vi "Old - Move Straight.vi"(6 "Angle Reduction Factor":dbl, 8 "error in (no error)":errorcluster, 9 "Encoder Reduction Factor":dbl, 10 "Ref-Nums":T1, 11 "Encoder Distance":dbl=-3600.0 format="%#_13g") -> (0 "error out":errorcluster)   [LabVIEW 2017]
uses:
  <vilib>/Rock Robotics/WPI/ThirdParty/Phoenix-LabVIEW/Motor Controller/Get/CTRE_Phoenix_MotorController_GetGeneralStatus.vi
  <vilib>/Rock Robotics/WPI/ThirdParty/Phoenix-LabVIEW/Motor Controller/Get/CTRE_Phoenix_MotorController_GetOutputCurrent_Enhanced.vi
panel:
  in  "Reduction Factor 3":dbl
  in  "Encoder Distance 3":dbl=-3600.0 format="%#_13g"
  in  "Reduction Factor 2":dbl
  in  "Encoder Distance 2":dbl=-3600.0 format="%#_13g"
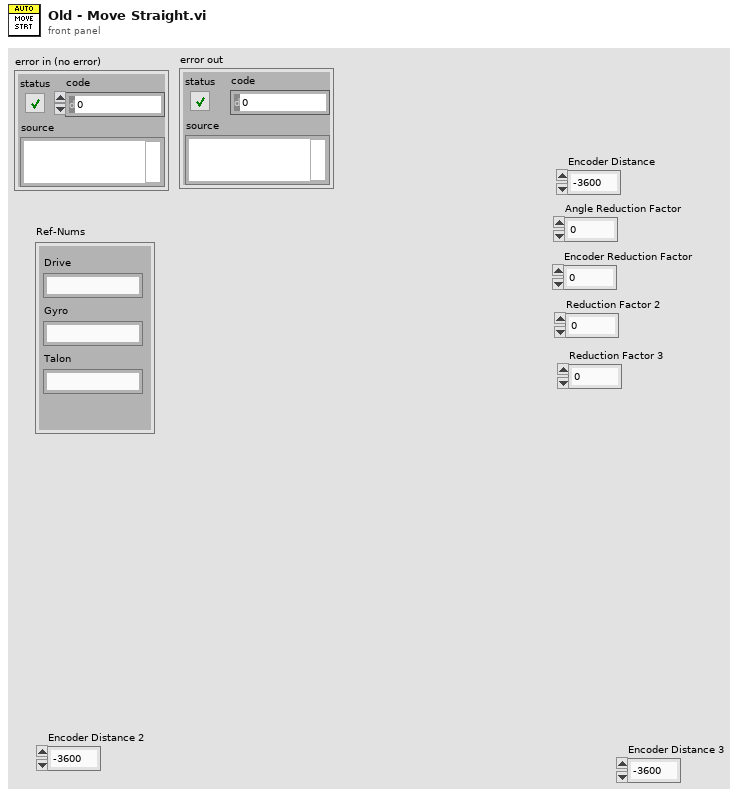
[diagram p1: front panel]
types:
  T1 = cluster{"Drive":string, "Gyro":string, "Talon":string}
  T2 = typedef "WPI_CANTalonSRX_GlobalStatus.ctl" = cluster{"Applied Throttle":dbl, "Module Enabled":bool, "CAN Error":errorcluster, "Closed Loop Error":dbl, "Forward Limit Switch Closed":bool, "Reverse Limit Switch Closed":bool, "Sensor Position":dbl, "Sensor Velocity":dbl, "Current":dbl, "Sticky Fault - Over Temp":bool, "Sticky Fault - Under Voltage":bool, "Sticky Fault - Forward Limit":bool, "Sticky Fault - Reverse Limit":bool, "Sticky Fault - Forward Soft Limit":bool, "Sticky Fault - Reverse Soft Limit":bool, "Brake is Enabled":bool, "Encoder Position":dbl, "Encoder Velocity":dbl, "Encoder Index Count":dbl, "Encoder A Pin State":bool, "Encoder B Pin State":bool, "Encoder Index Pin State":bool, "Analog In":dbl, "Analog In Velocity":dbl, "Temperature (C)":dbl, "Battery Voltage":dbl, "Control 5 Is Supported":bool, "Current Profile Slot Select":dbl, "Pos Div 8":bool, "Vel Div 4":bool, "Pulse Width Position":i32, "Pulse Width Velocity":i32, "Pulse Width Rise To Rise (us)":i32, "Pulse Width Rise To Fall (us)":i32, "Mot Prof Active Is Under Run":bool, "Mot Prof Active Has Under Run":bool, "Mot Prof Active Is Last":bool, "Mot Prof Active Velocity Only":bool, "Mot Prof Active Is Valid":bool, "Mot Prof Buffer Is Full":bool, "Mot Prof Active Profile Slot Select":i32, "Mot Prof NextID":i32, "Mot Prof Count":i32, "Mot Prof Active Velocity":dbl, "Mot Prof Active Position":dbl, "Mot Prof Output Enable":i32}
  T3 = typedef "WPI_MotorControlDeviceRef.ctl" = cluster{"DeviceStatus":errorcluster, "Type":T4, "PWM":cluster{"PWM Channel":T5, "DeadBand":T6}, "CAN":cluster{"Device Number":u8, "SetOutput VI Ref":variant, "GetOutput VI Ref":variant, "Enable VI Ref":variant, "Disable VI Ref":variant, "Data":variant}, "Invert":bool, "DIO PWM":cluster{"PWM \"Enable\" Channel":T5, "DIOChannel":T7, "PWM Rate":dbl}}
  T4 = typedef "WPI_MotorControlType.ctl" = enum16{"PWM", "CAN", "DIO PWM"}
  T5 = typedef "FPGA_DIOPWMChannel.ctl" = enum8{"PWM 0", "PWM 1", "PWM 2", "PWM 3", "PWM 4", "PWM 5", "PWM 6", "PWM 7", "PWM 8", "PWM 9", "PWM MXP 0", "PWM MXP 1", "PWM MXP 2", "PWM MXP 3", "PWM MXP 4", "PWM MXP 5", "PWM MXP 6", "PWM MXP 7", "PWM MXP 8", "PWM MXP 9", "Invalid"}
  T6 = typedef "WPI_PWMDeadband.ctl" = cluster{"Name":string, "maxPositivePwm":i32, "minPositivePwm":i32, "centerPwm":i32, "maxNegativePwm":i32, "minNegativePwm":i32, "angularRange":u16}
  T7 = typedef "FPGA_DIOChannel.ctl" = enum8{"DIO 0", "DIO 1", "DIO 2", "DIO 3", "DIO 4", "DIO 5", "DIO 6", "DIO 7", "DIO 8", "DIO 9", "DIO MXP 0", "DIO MXP 1", "DIO MXP 2", "DIO MXP 3", "DIO MXP 4", "DIO MXP 5", "DIO MXP 6", "DIO MXP 7", "DIO MXP 8", "DIO MXP 9", "DIO MXP 10", "DIO MXP 11", "DIO MXP 12", "DIO MXP 13", "DIO MXP 14", "DIO MXP 15", "SPI Port CS1", "SPI Port CS2", "SPI Port CS3", "SPI Port MISO", "SPI Port MOSI", "Invalid"}
  T8 = typedef "WPI_GyroDevRef.ctl" = cluster{"DevStatus":errorcluster, "Analog Channel":T9, "Gain (VoltsPerDegree/Second)":dbl, "Gyro Type":enum16{"Analog", "XRS450"}, "Handle":i32, "SPI Bus":T10, "Device Found":bool, "Sample Rate":dbl, "Calibrate On Open":bool, "Offset":dbl}
  T9 = typedef "FPGA_AIChannel.ctl" = enum8{"AI 0", "AI 1", "AI 2", "AI 3", "AI MXP 0", "AI MXP 1", "AI MXP 2", "AI MXP 3", "Invalid"}
  T10 = typedef "spi_bus.ctl" = enum16{"SPI On-Board, CS0", "SPI On-Board, CS1", "SPI On-Board, CS2", "SPI On-Board, CS3", "SPI MXP", "Invalid"}
  T11 = typedef "WPI_RobotDriveDevRef.ctl" = cluster{"DevStatus":errorcluster, "Motors[]":T3[], "Square Inputs":bool, "Max Output":dbl}
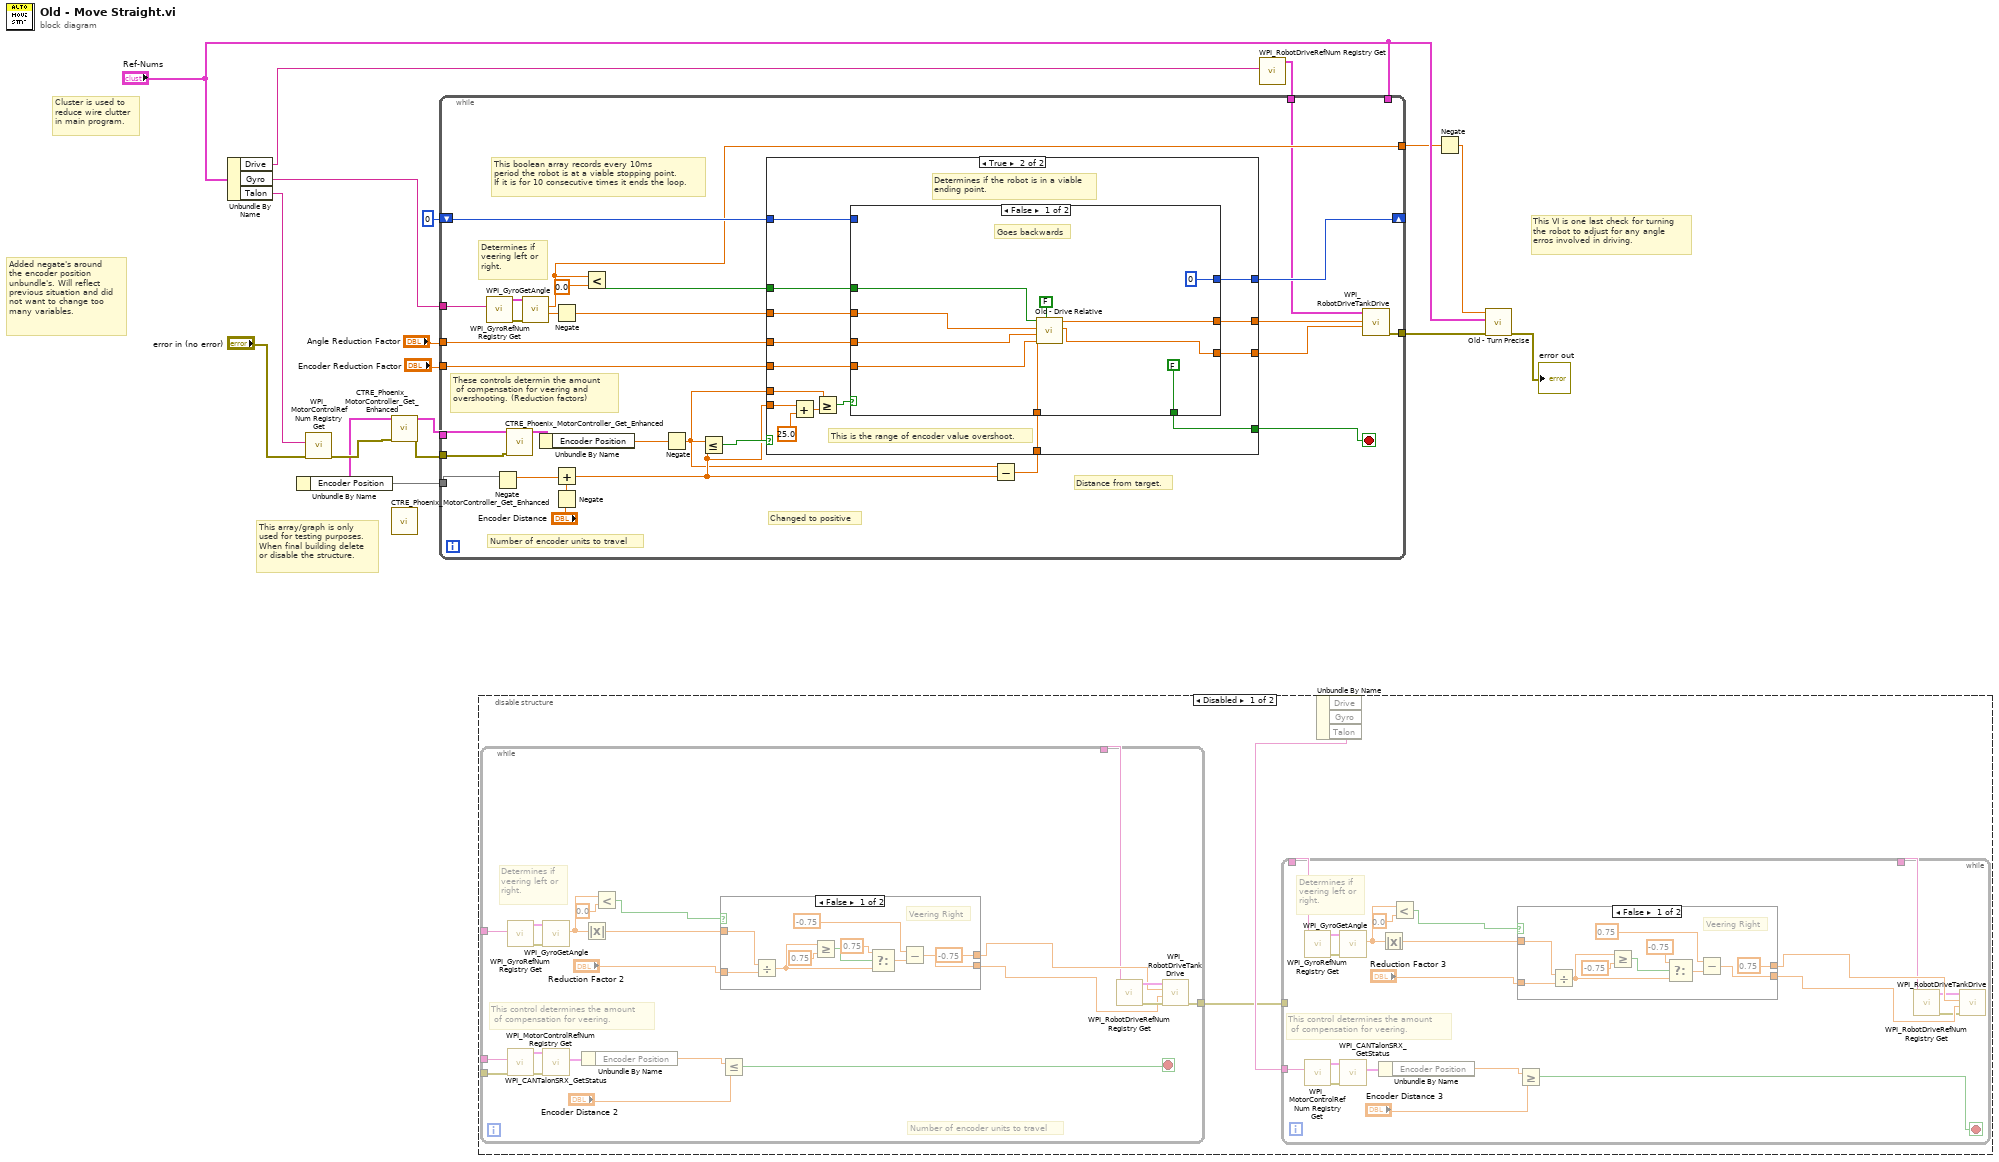
[diagram p0: block diagram]
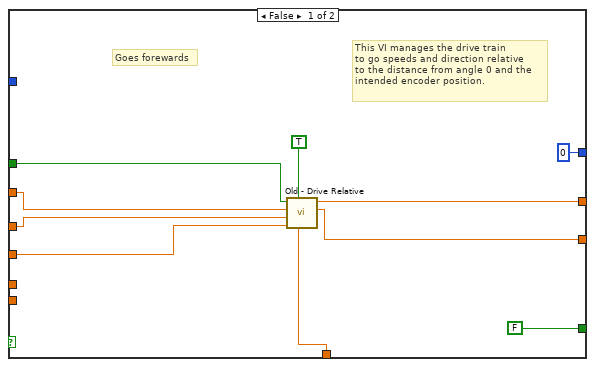
[diagram p2: hidden frame]
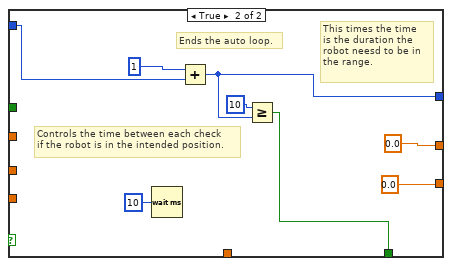
[diagram p3: hidden frame]
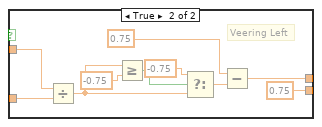
[diagram p4: hidden frame]
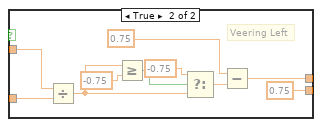
[diagram p5: hidden frame]
diagram:
  # "Added negate's around\nthe encoder position \nunbundle's. Will reflect\nprevious situation and did\nnot want to change too \nmany variables."
  # "This VI is one last check for turning\nthe robot to adjust for any angle \nerros involved in driving."
  # "This array/graph is only\nused for testing purposes.\nWhen final building delete\nor disable the structure."
  # "Cluster is used to\nreduce wire clutter\nin main program."
  n1 = Unbundle By Name("Ref-Nums") -> ("Drive"=w8:string, "Gyro"=w18:string, "Talon"=w11:string)
  n2 = Unbundle By Name() -> (w1:T2, "Encoder Position"=w9)
  n3 = call <vilib>:"WPI_MotorControlRefNum Registry Get.vi"("error in (no error)"="error in (no error)", "refnum name"=w11) -> ("error out"=w3:errorcluster)  [unwired: 8 in, 1 out]
  n4 = call-poly <vilib>:"CTRE_Phoenix_MotorController_Get_Enhanced.vi"("PhoenixMotorControlDevRef"=w1, "error in"=w3) -> ("PhoenixMotorControlDevRef"=w4:T3, "error out"=w2:errorcluster)  [unwired: 11 in, 1 out]
  n5 = call-poly <vilib>:"CTRE_Phoenix_MotorController_Get_Enhanced.vi"() -> ()  [unwired: 10 in, 6 out]
  n6 = disable-structure shown="Disabled" {
    frame Disabled {
      n7 = while {
        tunnel: _ -> [w74]
        tunnel: _ -> [w73]
        tunnel: [w72] -> w19
        tunnel: [w71] -> w21
        tunnel: [w66] -> w20
        stop <- w65 stop-if-true
        # "Determines if \nveering left or \nright."
        # "This control determines the amount\n of compensation for veering."
        # "Number of encoder units to travel"
        n8 = call <vilib>:"WPI_GyroRefNum Registry Get.vi"("refnum name"=w73) -> ("error out"=w81:errorcluster, "GyroDevRef"=w82:T8)  [unwired: 9 in]
        n9 = call <vilib>:"WPI_MotorControlRefNum Registry Get.vi"("error in (no error)"=w74, "refnum name"=w72) -> ("error out"=w75:errorcluster, "MotorControlDevRef"=w76:T3)  [unwired: 8 in]
        n10 = call <vilib>:"WPI_GyroGetAngle.vi"("error in"=w81, "GyroDevRef"=w82) -> ("Angle"=w80:dbl)  [unwired: 5 in, 4 out]
        n11 = call <vilib>:"WPI_CANTalonSRX_GetStatus.vi"("error in (no error)"=w75, "CAN Talon SRX Ref"=w76) -> ("Talon SRX Status"=w77:T2)  [unwired: 7 in, 2 out]
        n12 = Unbundle By Name(w77) -> ("Encoder Position"=w70:dbl)
        n13 = Absolute Value(x=w80) -> (abs(x)=w84:dbl)
        n14 = Less?(x=w80, y=0.0) -> (x < y?=w85:bool)
        n15 = case shown="False" w85 {
          tunnel: [-0.75 w100] -> w68
          tunnel: [w89 0.75] -> w67
          tunnel: w84 -> [w88 w98]
          tunnel: "Reduction Factor 2" -> [w87 w97]
          frame False {
            # "Veering Right"
            n16 = Divide(x=w88, y=w87) -> (x/y=w91:dbl)
            n17 = Greater Or Equal?(x=w91, y=0.75) -> (x >= y?=w95:bool)
            n18 = Select(t=0.75, s=w95, f=w91) -> (s? t:f=w92:dbl)
            n19 = Subtract(x=-0.75 ("y"), y=w92) -> (x-y=w89:dbl)
          }
          frame True {
            # "Veering Left"
            n20 = Divide(x=w98, y=w97) -> (x/y=w101:dbl)
            n21 = Greater Or Equal?(x=w101, y=-0.75) -> (x >= y?=w105:bool)
            n22 = Select(t=-0.75, s=w105, f=w101) -> (s? t:f=w102:dbl)
            n23 = Subtract(x=0.75 ("y"), y=w102) -> (x-y=w100:dbl)
          }
        }
        n24 = Less Or Equal?(x=w70, y="Encoder Distance 2") -> (x <= y?=w65:bool)
        n25 = call <vilib>:"WPI_RobotDriveRefNum Registry Get.vi"("refnum name"=w66) -> ("error out"=w79:errorcluster, "RobotDriveDevRef"=w78:T11)  [unwired: 9 in]
        n26 = call <vilib>:"WPI_RobotDriveTankDrive.vi"("error in (no error)"=w79, "Right axis value"=w67, "Left axis value"=w68, "RobotDriveDevRef"=w78) -> ("error out"=w71:errorcluster)  [unwired: 5 in, 2 out]
      }
      n27 = Unbundle By Name() -> ("Talon"=w24:string)  [unwired: 1 in, 2 out]
      n28 = while {
        tunnel: w21 -> [_]
        tunnel: [w27] -> w22
        tunnel: [w26] -> w23
        tunnel: w24 -> [w25]
        stop <- w28 stop-if-true
        # "Determines if \nveering left or \nright."
        # "This control determines the amount\n of compensation for veering."
        n29 = call <vilib>:"WPI_GyroRefNum Registry Get.vi"("refnum name"=w26) -> ("error out"=w34:errorcluster, "GyroDevRef"=w33:T8)  [unwired: 9 in]
        n30 = call <vilib>:"WPI_MotorControlRefNum Registry Get.vi"("refnum name"=w25) -> ("error out"=w40:errorcluster, "MotorControlDevRef"=w39:T3)  [unwired: 9 in]
        n31 = call <vilib>:"WPI_GyroGetAngle.vi"("error in"=w34, "GyroDevRef"=w33) -> ("Angle"=w35:dbl)  [unwired: 5 in, 4 out]
        n32 = call <vilib>:"WPI_CANTalonSRX_GetStatus.vi"("error in (no error)"=w40, "CAN Talon SRX Ref"=w39) -> ("Talon SRX Status"=w38:T2)  [unwired: 7 in, 2 out]
        n33 = Unbundle By Name(w38) -> ("Encoder Position"=w41:dbl)
        n34 = Absolute Value(x=w35) -> (abs(x)=w31:dbl)
        n35 = Less?(x=w35, y=0.0) -> (x < y?=w30:bool)
        n36 = case shown="False" w30 {
          tunnel: [0.75 w58] -> w43
          tunnel: [w47 0.75] -> w44
          tunnel: w31 -> [w46 w56]
          tunnel: "Reduction Factor 3" -> [w45 w55]
          frame False {
            # "Veering Right"
            n37 = Divide(x=w46, y=w45) -> (x/y=w49:dbl)
            n38 = Greater Or Equal?(x=w49, y=-0.75) -> (x >= y?=w53:bool)
            n39 = Select(t=-0.75, s=w53, f=w49) -> (s? t:f=w50:dbl)
            n40 = Subtract(x=0.75 ("y"), y=w50) -> (x-y=w47:dbl)
          }
          frame True {
            # "Veering Left"
            n41 = Divide(x=w56, y=w55) -> (x/y=w59:dbl)
            n42 = Greater Or Equal?(x=w59, y=-0.75) -> (x >= y?=w63:bool)
            n43 = Select(t=-0.75, s=w63, f=w59) -> (s? t:f=w60:dbl)
            n44 = Subtract(x=0.75 ("y"), y=w60) -> (x-y=w58:dbl)
          }
        }
        n45 = Greater Or Equal?(x=w41, y="Encoder Distance 3") -> (x >= y?=w28:bool)
        n46 = call <vilib>:"WPI_RobotDriveRefNum Registry Get.vi"("refnum name"=w27) -> ("error out"=w36:errorcluster, "RobotDriveDevRef"=w37:T11)  [unwired: 9 in]
        n47 = call <vilib>:"WPI_RobotDriveTankDrive.vi"("error in (no error)"=w36, "Right axis value"=w44, "Left axis value"=w43, "RobotDriveDevRef"=w37) -> ()  [unwired: 5 in, 3 out]
      }
    }
    frame Enabled {
    }
  }
  n48 = call <vilib>:"WPI_RobotDriveRefNum Registry Get.vi"("refnum name"=w8) -> ("RobotDriveDevRef"=w7:T11)  [unwired: 9 in, 1 out]
  n49 = while {
    tunnel: w18 -> [w131]
    tunnel: w4 -> [w107]
    tunnel: [w130] -> w13
    shift-right: [w125] -> _
    shift-left: 0 -> [w124]
    tunnel: [w122] -> w15
    tunnel: "Ref-Nums" -> [_]
    tunnel: w9 -> [w110]
    tunnel: w7 -> [w120]
    tunnel: "Angle Reduction Factor" -> [w119]
    tunnel: "Encoder Reduction Factor" -> [w118]
    tunnel: w2 -> [w108]
    stop <- w128 stop-if-true
    # "Changed to positive"
    # "Distance from target."
    # "This boolean array records every 10ms\nperiod the robot is at a viable stopping point.\nIf it is for 10 consecutive times it ends the loop."
    # "Determines if \nveering left or \nright."
    # "These controls determin the amount\n of compensation for veering and \novershooting. (Reduction factors)"
    # "Number of encoder units to travel"
    n50 = call <vilib>:"WPI_GyroRefNum Registry Get.vi"("refnum name"=w131) -> ("error out"=w132:errorcluster, "GyroDevRef"=w133:T8)  [unwired: 9 in]
    n51 = Negate(x=w110) -> (-x=w111:dbl)
    n52 = call-poly <vilib>:"CTRE_Phoenix_MotorController_Get_Enhanced.vi"("PhoenixMotorControlDevRef"=w107, "error in"=w108) -> ("PhoenixMotorControlDevRef"=w109:T3)  [unwired: 8 in, 5 out]
    n53 = call <vilib>:"WPI_GyroGetAngle.vi"("error in"=w132, "GyroDevRef"=w133) -> ("Angular Rate"=w116:dbl, "Angle"=w122:dbl)  [unwired: 5 in, 3 out]
    n54 = Unbundle By Name(w109) -> ("Encoder Position"=w114:dbl)
    n55 = Negate(x=w116) -> (-x=w117:dbl)
    n56 = Negate(x="Encoder Distance") -> (-x=w113:dbl)
    n57 = Add(x=w111, y=w113) -> (x+y=w121:dbl)
    n58 = Less?(x=w122, y=0.0) -> (x < y?=w134:bool)
    n59 = Negate(x=w114) -> (-x=w115:dbl)
    n60 = Less Or Equal?(x=w115, y=w121) -> (x <= y?=w129:bool)
    n61 = Subtract(x=w115, y=w121) -> (x-y=w123:dbl)
    n62 = case shown="True" w129 {
      tunnel: w134 -> [w145 w160]
      tunnel: w117 -> [w144 w159]
      tunnel: w119 -> [w143 w158]
      tunnel: w115 -> [_ w156]
      tunnel: [w142 w152] -> w127
      tunnel: [w141 w151] -> w126
      tunnel: [FALSE w153] -> w128
      tunnel: [0 w150] -> w125
      tunnel: w124 -> [_ w149]
      tunnel: w121 -> [_ w148]
      tunnel: w123 -> [w138 w146]
      tunnel: w118 -> [w137 w147]
      frame False {
        # "This VI manages the drive train\nto go speeds and direction relative\nto the distance from angle 0 and the\nintended encoder position."
        # "Goes forewards"
        n63 = call "Old - Drive Relative.vi"("Distance From Target"=w138, "Encoder Direction"=TRUE, "Encoder Reduction Factor"=w137, "Angle Reduction Factor"=w143, "Angle"=w144, "Angle Direction"=w145) -> ("Right Power"=w141:dbl, "Left Power"=w142:dbl)  [unwired: 4 in]
      }
      frame True {
        # "This is the range of encoder value overshoot."
        # "Determines if the robot is in a viable\nending point."
        n64 = Add(x=w148, y=25.0) -> (x+y=w154:dbl)
        n65 = Greater Or Equal?(x=w156, y=w154) -> (x >= y?=w157:bool)
        n66 = case shown="False" w157 {
          tunnel: w160 -> [w168 _]
          tunnel: w159 -> [w167 _]
          tunnel: w158 -> [w166 _]
          tunnel: [FALSE w171] -> w153
          tunnel: [w162 0.0] -> w152
          tunnel: [w163 0.0] -> w151
          tunnel: [0 w173] -> w150
          tunnel: w149 -> [_ w174]
          tunnel: w147 -> [w165 _]
          tunnel: w146 -> [w164 _]
          frame False {
            # "Goes backwards"
            n67 = call "Old - Drive Relative.vi"("Distance From Target"=w164, "Encoder Direction"=FALSE, "Encoder Reduction Factor"=w165, "Angle Reduction Factor"=w166, "Angle"=w167, "Angle Direction"=w168) -> ("Right Power"=w163:dbl, "Left Power"=w162:dbl)  [unwired: 4 in]
          }
          frame True {
            # "This times the time\nis the duration the \nrobot neesd to be in \nthe range."
            # "Controls the time between each check\nif the robot is in the intended position."
            # "Ends the auto loop."
            n68 = Wait (ms)(milliseconds to wait=u32 10) -> ()  [unwired: 1 out]
            n69 = Add(x=1, y=w174) -> (x+y=w173:i32)
            n70 = Greater Or Equal?(x=10, y=w173) -> (x >= y?=w171:bool)
          }
        }
      }
    }
    n71 = call <vilib>:"WPI_RobotDriveTankDrive.vi"("Right axis value"=w126, "Left axis value"=w127, "RobotDriveDevRef"=w120) -> ("error out"=w130:errorcluster)  [unwired: 6 in, 2 out]
  }
  n72 = Negate(x=w15) -> (-x=w14:dbl)
  n73 = call "Old - Turn Precise.vi"("error in (no error)"=w13, "Ref-Nums"="Ref-Nums", "Angle"=w14) -> ("error out"=→"error out":errorcluster)  [unwired: 8 in]
